vi "SP24_CL_Framework_0.vi"() -> ()   [LabVIEW 2023]
uses:
  <vilib>/Analysis/3filter.llb/Filter Passband Type.ctl
  LVLib/SADI_FW3.lvlib
  <vilib>/ptbypt/NI_PtbyPt.lvlib
  <vilib>/Analysis/NI_AALBase.lvlib
panel:
  in  "Couts/rev":dbl=3704.0
  in  "Tab Control":T1(tab)=enum."Stuff you need to use"
  in  "Latest?":bool=TRUE
  out "SADIs Connected":u32=1
  in  "instance":i32
  in  "Loop Frequency":u16=30000 min=1
  out "MSG CNT":u32=7246531
  in  "Mode Select":T2(ring)=enum."daqMode_pendulum"
  in  "Encoder Pin Location 1":u16(ring)=2 items=["D0"=0, "D1"=1, "D2"=2, "D3"=3, "D4"=4, "D5"=5, "D6"=6, "D8"=8, "D9"=9, "D10"=10, "D11"=11]
  in  "Encoder Pin Location 0":u16(ring) items=["D0"=0, "D1"=1, "D2"=2, "D3"=3, "D4"=4, "D5"=5, "D6"=6, "D8"=8, "D9"=9, "D10"=10, "D11"=11]
  in  "OutputPinMsk":u16=240 format="%x"
  in  "servoEnableMask":u8 format="%x"
  in  "motorEnableMask":u8 format="%x"
  out "Setup Valid":bool=TRUE
  out "Stopped":bool=TRUE
  in  "Output Units":enum16{"Degrees", "Radians"}(ring)
  out "PendEncValMax":u16=500
  in  "ADC GAIN 0":u16(ring)=2 items=["Range_CH_OFF_msk"=0, "Range_pm_10_24_msk"=1, "Range_pm_05_12_msk"=2, "Range_pm_02_56_msk"=3, "Range_pm_01_28_msk"=4, "Range_pm_00_64_msk"=5, "Range_10_24_msk"=9, "Range_05_12_msk"=10, "Range_02_56_msk"=11, "Range_01_28_msk"=12]
  in  "ADC GAIN 3":u16(ring)=2 items=["Range_CH_OFF_msk"=0, "Range_pm_10_24_msk"=1, "Range_pm_05_12_msk"=2, "Range_pm_02_56_msk"=3, "Range_pm_01_28_msk"=4, "Range_pm_00_64_msk"=5, "Range_10_24_msk"=9, "Range_05_12_msk"=10, "Range_02_56_msk"=11, "Range_01_28_msk"=12]
  in  "ADC GAIN 2":u16(ring)=2 items=["Range_CH_OFF_msk"=0, "Range_pm_10_24_msk"=1, "Range_pm_05_12_msk"=2, "Range_pm_02_56_msk"=3, "Range_pm_01_28_msk"=4, "Range_pm_00_64_msk"=5, "Range_10_24_msk"=9, "Range_05_12_msk"=10, "Range_02_56_msk"=11, "Range_01_28_msk"=12]
  in  "ADC GAIN 1":u16(ring)=2 items=["Range_CH_OFF_msk"=0, "Range_pm_10_24_msk"=1, "Range_pm_05_12_msk"=2, "Range_pm_02_56_msk"=3, "Range_pm_01_28_msk"=4, "Range_pm_00_64_msk"=5, "Range_10_24_msk"=9, "Range_05_12_msk"=10, "Range_02_56_msk"=11, "Range_01_28_msk"=12]
  out "FT_ERROR_ENUM":T3(ring)=enum."FT_INVALID_HANDLE"
  out "Loop Time (ms)":dbl=0.48749999950814527 format="%.6f"
  in  "Encoder Resolution 0":u16=360
  in  "Encoder Resolution 1":u16=360
  out "PendEncValMin":u16=10000
  out "Software Version":dbl=3.024 format="%_6g"
  out "Firmware Version":sgl=3.41
  out "Motor Rotation Counts":i32=31626
  out "Motor Velocity":i32=5788
  in  "Cutoff freq: fl":dbl=40.0 format="%0.3f"
  in  "Sampling freq: fs":dbl=2000.0
  in  "initialize":bool
  out "Filtered Platen Rotation Angle":dbl=3294.999499487255 format="%0.2f"
  out "Platen Velocity":dbl=-3.1364198416679514
  out "Total Angle":dbl=3295.4967602591796
  in  "Zero":bool
  in  "Amplitude":dbl=350.0
  in  "Turn On Command":dbl=65.0
  in  "Frequency":dbl=20.0
  in  "Sine (L)/Square (R)":bool
  in  "Enable Motor":bool=TRUE
  in  "Stop":bool=TRUE
  in  "Desired Loop \nTime (ms)":dbl=0.5
  out "Actual Loop \nTime (ms)":dbl=0.500105999999505
  out "Elapsed \nTime (s)":dbl=241.6297153000005
  out "Segments Saved":u32=1
  in  "Save Data?":bool
  out "Platen Rotation Graph":dbl[](graph)=[3294.999499487255]
  out "Platen Vel Graph":dbl[](graph)=[-3.1364198416679514]
  out "Command Signal Graph":dbl[](graph)=[-176.84915368007944]
  out "Command Signal":dbl=-176.84915368007944
  out "Read Call Error Out":u16(ring)=32768 items=["SADI_RESET (FT_OK)"=0, "FT_INVALID_HANDLE"=1, "FT_DEVICE_NOT_FOUND"=2, "FT_DEVICE_NOT_OPENED"=3, "FT_IO_ERROR"=4, "FT_INSUFFICIENT_RESOURCES"=5, "FT_OTHER_ERROR"=18, "FT_NOT_SUPPORTED"=17, "DATA_RECEIVED"=32768, "NO_DATA_AVAIL"=32769, "NO_SADI"=32770]
  out "SADI State":T4(ring)=enum."Run_state"
  # "Platen Rotation & Velocity"
  # "Signal Generator"
  # "Butterworth Filter Settings"
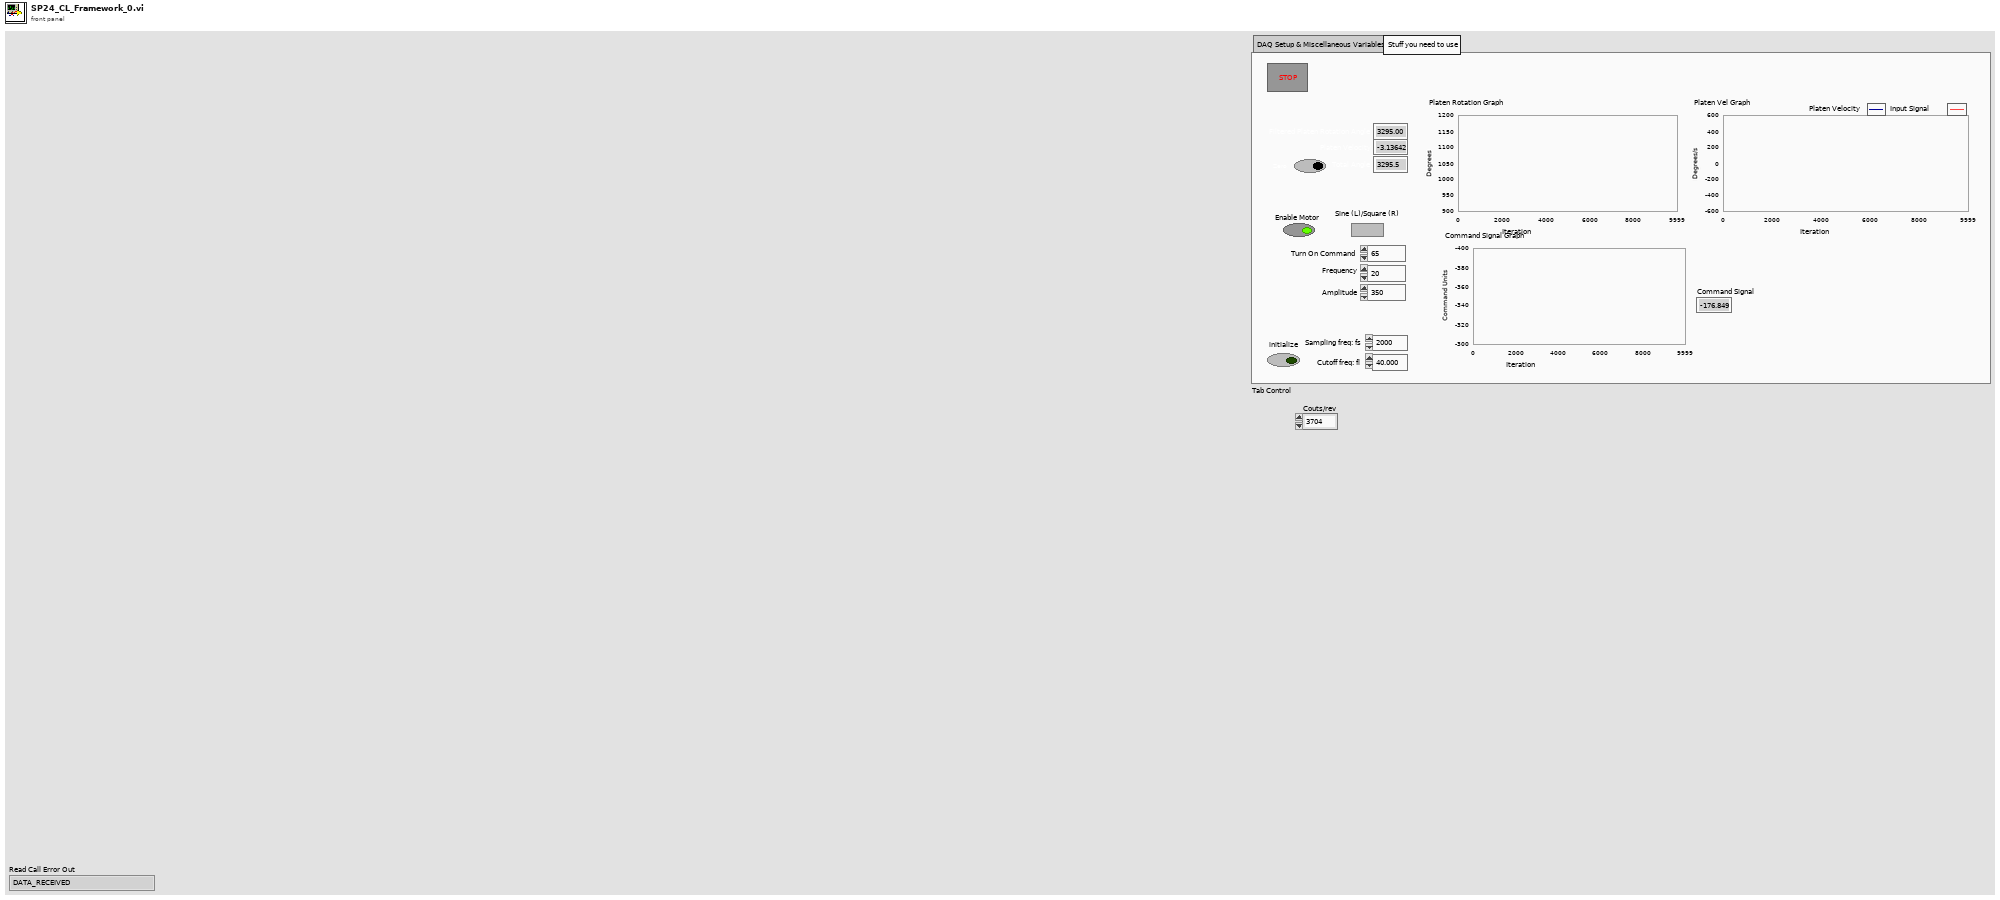
[diagram p1: front panel]
types:
  T1 = enum32{"DAQ Setup & Miscellaneous Variables", "Stuff you need to use"}
  T2 = enum16{"daqMode_unassigned", "daqMode_generic", "daqMode_pendulum", "daqMode_mom"}
  T3 = enum32{"FT_OK", "FT_INVALID_HANDLE", "FT_DEVICE_NOT_FOUND", "FT_DEVICE_NOT_OPENED", "FT_IO_ERROR", "FT_INSUFFICIENT_RESOURCES", "FT_INVALID_PARAMETER", "FT_INVALID_BAUD_RATE", "FT_DEVICE_NOT_OPENED_FOR_ERASE", "FT_DEVICE_NOT_OPENED_FOR_WRITE", "FT_FAILED_TO_WRITE_DEVICE", "FT_EEPROM_READ_FAILED", "FT_EEPROM_WRITE_FAILED", "FT_EEPROM_ERASE_FAILED", "FT_EEPROM_NOT_PRESENT", "FT_EEPROM_NOT_PROGRAMMED", "FT_INVALID_ARGS", "FT_NOT_SUPPORTED", "FT_OTHER_ERROR", "FT_DEVICE_LIST_NOT_READY"}
  T4 = enum32{"NotOpened_state", "Opened_state", "Ready_state", "Setup_state", "InitSent_state", "Start_initiated_state", "Run_state", "StopInitiated_state", "Stopped_state"}
  T5 = typedef "NI_AALBase.lvlib/Filter Passband Type.ctl" = enum32{"Lowpass", "Highpass", "Bandpass", "Bandstop"}
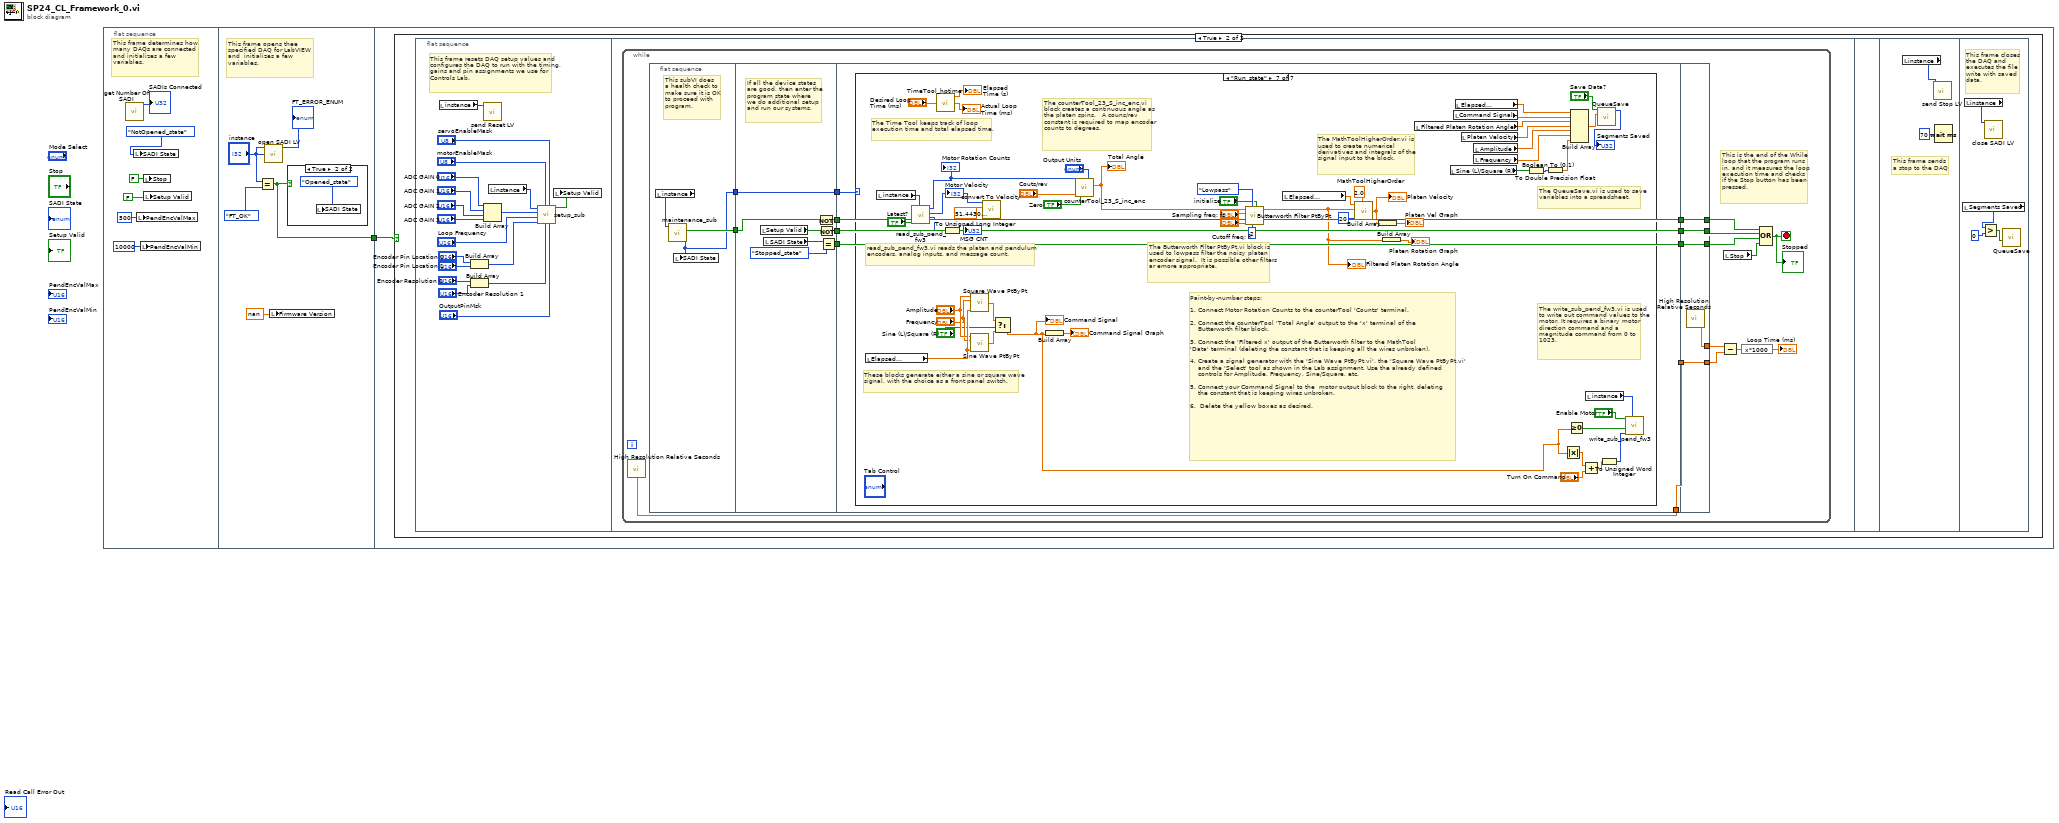
[diagram p0: block diagram]
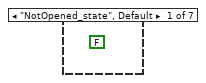
[diagram p4: hidden frame]
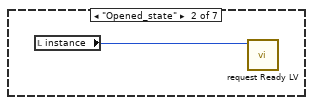
[diagram p5: hidden frame]
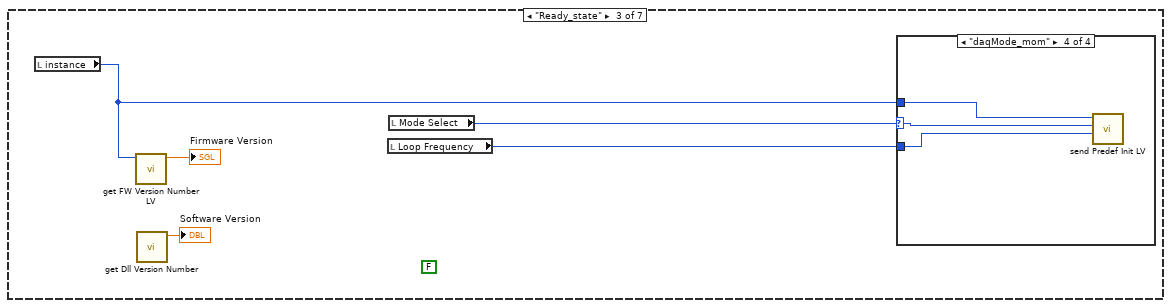
[diagram p6: hidden frame]
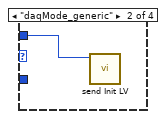
[diagram p8: hidden frame]
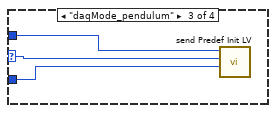
[diagram p9: hidden frame]
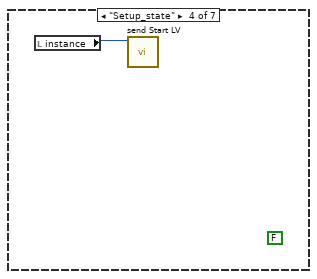
[diagram p10: hidden frame]
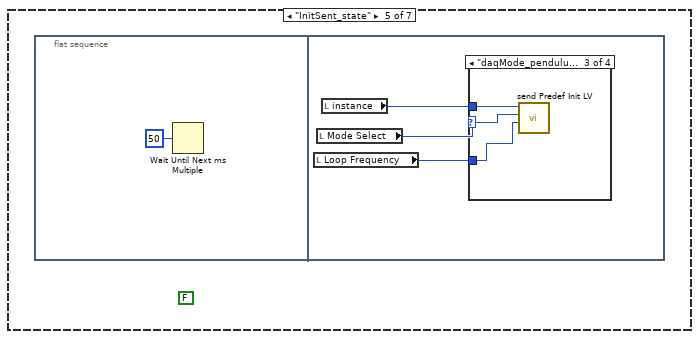
[diagram p11: hidden frame]
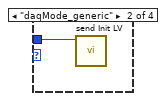
[diagram p13: hidden frame]
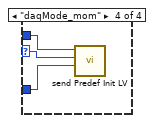
[diagram p14: hidden frame]
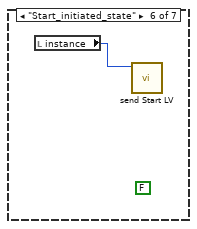
[diagram p15: hidden frame]
diagram:
  n1 = flat-sequence {
    tunnel: [w10] -> w1
    tunnel: w1 -> [w14]
    frame #0 {
      # "This frame determines how many DAQs are connected and initializes a few variables."
      n2 = call "get Number Of SADI.vi"() -> ("function return"=→"SADIs Connected":u32)  [unwired: 11 in]
      n3 = local write "SADI State"(T4."NotOpened_state" ("SADI State")) -> ()
      n4 = local write "PendEncValMax"(u16 500 ("PendEncValMax")) -> ()
      n5 = local write "PendEncValMin"(u16 10000 ("PendEncValMin")) -> ()
      n6 = local write "Stop"(FALSE ("Stop")) -> ()
      n7 = local write "Setup Valid"(FALSE ("Setup Valid")) -> ()
    }
    frame #1 {
      # "This frame opens thee specified DAQ for LabVIEW and  initializes a few variables."
      n8 = Equal?(x="instance", y=T3."FT_OK" ("FT_ERROR_ENUM 2")) -> (x = y?=w10:bool)
      n9 = call "open SADI LV.vi"("deviceNumber"="instance", "instance"="instance") -> ("function return"=→"FT_ERROR_ENUM":u32)  [unwired: 9 in]
      n10 = local write "Firmware Version"(nan ("Firmware Version")) -> ()
      n11 = case shown="True" w10 {
        frame False {
        }
        frame True {
          n12 = local write "SADI State"(T4."Opened_state" ("SADI State 2")) -> ()
        }
      }
    }
    frame #2 {
      n13 = case shown="True" w14 {
        frame False {
        }
        frame True {
          n14 = flat-sequence {
            frame #0 {
              # "This frame resets DAQ setup values and configures the DAQ to run with the timing, gains and pin assignments we use for Controls Lab."
              n15 = local read "instance"() -> (w16:i32)
              n16 = Build Array("Encoder Pin Location 0", "Encoder Pin Location 1") -> (w26:u16[])
              n17 = Build Array("Encoder Resolution 0", "Encoder Resolution 1") -> (w23:u16[])
              n18 = Build Array("ADC GAIN 0", "ADC GAIN 1", "ADC GAIN 2", "ADC GAIN 3") -> (w28:u16[])
              n19 = call "send Reset LV.vi"("instance"=w16) -> ()  [unwired: 11 in]
              n20 = local read "instance"() -> (w17:i32)
              n21 = call "setup_sub.vi"("OutputPinMsk"="OutputPinMsk", "servoEnableMask"="servoEnableMask", "ENC_RES_Array"=w23, "motorEnableMask"="motorEnableMask", "pinLocation_Array"=w26, "Loop Frequency"="Loop Frequency", "ADC_Settings"=w28, "instance"=w17) -> ("Success?"=w18:bool)  [unwired: 3 in]
              n22 = local write "Setup Valid"(w18) -> ()
            }
            frame #1 {
              n23 = while {
                stop <- w47 stop-if-true
                # "This is the end of the While \nloop that the program runs\nin, and it measures the loop\nexecution time and checks\nif the Stop button has been\npressed."
                n24 = call <vilib>:"High Resolution Relative Seconds.vi"() -> ("relative seconds"=w35:dbl)
                n25 = flat-sequence {
                  tunnel: [w55] -> w52
                  tunnel: [w53] -> w33
                  tunnel: w52 -> [w60]
                  tunnel: [w59] -> w46
                  tunnel: [w58] -> w45
                  tunnel: [w57] -> w44
                  tunnel: [w56] -> w34
                  tunnel: w33 -> [w56]
                  tunnel: w46 -> [w68]
                  tunnel: w45 -> [w67]
                  tunnel: w44 -> [w66]
                  tunnel: [w68] -> w43
                  tunnel: [w67] -> w42
                  tunnel: [w66] -> w41
                  tunnel: [w65] -> w39
                  tunnel: w35 -> [w65]
                  tunnel: w34 -> [w64]
                  tunnel: [w150] -> w49
                  tunnel: [w151] -> w50
                  tunnel: [w152] -> w51
                  tunnel: w43 -> [w152]
                  tunnel: w42 -> [w151]
                  tunnel: w41 -> [w150]
                  tunnel: [w149] -> w40
                  tunnel: w39 -> [w148]
                  tunnel: [w148] -> w38
                  frame #0 {
                    # "This subVI does\na health check to\nmake sure it is OK\nto proceed with\nprogram."
                    n26 = local read "instance"() -> (w54:i32)
                    n27 = call "maintenance_sub.vi"("Instance"=w54) -> ("SADI State"=w53:T4, "FT_OK?"=w55:bool)  [unwired: 8 in, 1 out]
                    n28 = local write "SADI State"(w53) -> ()
                  }
                  frame #1 {
                    # "If all the device states\nare good, then enter the\nprogram state where\nwe do additional setup\nand run our systems."
                    n29 = local read "Setup Valid"() -> (w63:bool)
                    n30 = local read "SADI State"() -> (w61:T4)
                    n31 = Not(x=w60) -> (.not. x?=w59:bool)
                    n32 = Not(x=w63) -> (.not. x?=w58:bool)
                    n33 = Equal?(x=w61, y=T4."Stopped_state") -> (x = y?=w57:bool)
                  }
                  frame #2 {
                    n34 = case shown="\"Run_state\"" w64 {
                      frame "NotOpened_state", Default {
                        (unwired) FALSE ("dataToRead?")
                      }
                      frame "Opened_state" {
                        n35 = local read "instance"() -> (w69:i32)
                        n36 = call "request Ready LV.vi"("instance"=w69) -> ()  [unwired: 11 in]
                      }
                      frame "Ready_state" {
                        (unwired) FALSE ("dataToRead?")
                        n37 = local read "instance"() -> (w72:i32)
                        n38 = call "get FW Version Number LV.vi"("instance"=w72) -> ("function return"=→"Firmware Version":dbl)  [unwired: 10 in]
                        n39 = call "get Dll Version Number.vi"() -> ("function return"=→"Software Version":dbl)  [unwired: 11 in]
                        n40 = local read "Loop Frequency"() -> (w70:u16)
                        n41 = local read "Mode Select"() -> (w71:T2)
                        n42 = case shown="\"daqMode_mom\"" w71 {
                          selector: w71 -> [_ _ w77 w80]
                          tunnel: w72 -> [_ w75 w78 w81]
                          tunnel: w70 -> [_ _ w76 w79]
                          frame "daqMode_unassigned", Default {
                          }
                          frame "daqMode_generic" {
                            n43 = call "send Init LV.vi"("instance"=w75) -> ()  [unwired: 11 in]
                          }
                          frame "daqMode_pendulum" {
                            n44 = call "send Predef Init LV.vi"("freq"=w76, "selection"=w77, "instance"=w78) -> ()  [unwired: 9 in]
                          }
                          frame "daqMode_mom" {
                            n45 = call "send Predef Init LV.vi"("freq"=w79, "selection"=w80, "instance"=w81) -> ()  [unwired: 9 in]
                          }
                        }
                      }
                      frame "Setup_state" {
                        (unwired) FALSE ("dataToRead?")
                        n46 = local read "instance"() -> (w82:i32)
                        n47 = call "send Start LV.vi"("instance"=w82) -> ()  [unwired: 11 in]
                      }
                      frame "InitSent_state" {
                        (unwired) FALSE ("dataToRead?")
                        n48 = flat-sequence {
                          frame #0 {
                            n49 = Wait Until Next ms Multiple(millisecond multiple=u32 50) -> ()  [unwired: 1 out]
                          }
                          frame #1 {
                            n50 = local read "Loop Frequency"() -> (w84:u16)
                            n51 = local read "Mode Select"() -> (w85:T2)
                            n52 = local read "instance"() -> (w86:i32)
                            n53 = case shown="\"daqMode_pendulum\"" w85 {
                              selector: w85 -> [_ _ w90 w92]
                              tunnel: w86 -> [_ w87 w89 w93]
                              tunnel: w84 -> [_ _ w88 w91]
                              frame "daqMode_unassigned", Default {
                              }
                              frame "daqMode_generic" {
                                n54 = call "send Init LV.vi"("instance"=w87) -> ()  [unwired: 11 in]
                              }
                              frame "daqMode_pendulum" {
                                n55 = call "send Predef Init LV.vi"("freq"=w88, "selection"=w90, "instance"=w89) -> ()  [unwired: 9 in]
                              }
                              frame "daqMode_mom" {
                                n56 = call "send Predef Init LV.vi"("freq"=w91, "selection"=w92, "instance"=w93) -> ()  [unwired: 9 in]
                              }
                            }
                          }
                        }
                      }
                      frame "Start_initiated_state" {
                        (unwired) FALSE ("dataToRead?")
                        n57 = local read "instance"() -> (w94:i32)
                        n58 = call "send Start LV.vi"("instance"=w94) -> ()  [unwired: 11 in]
                      }
                      frame "Run_state" {
                        # "Paint-by-number steps:\n\n1. Connect Motor Rotation Counts to the counterTool 'Counts' terminal.\n\n2. Connect the counterTool 'Total Angle' output to the 'x' terminal of the \n    Butterworth filter block.\n\n3. Connect the 'FIltered x' output of the Butterworth filter to the MathTool \n'Data' terminal (deleting the constant that is keeping all the wires unbroken).\n\n4. Create a signal generator with the 'Sine Wave PtByPt.vi', the 'Square Wave PtByPt.vi'\n    and the 'Select' tool as shown in the Lab assignment. Use the already defined\n    controls for Amplitude, Frequency, Sine/Square, etc.\n\n5. Connect your Command Signal to the  motor output block to the right, deleting\n    the constant that is keeping wires unbroken.\n\n6.  Delete the yellow boxes as desired."
                        # "The counterTool_23_S_inc_enc.vi block creates a continuous angle as the platen spins.   A couns/rev constant is required to map encoder counts to degrees."
                        # "The write_sub_pend_fw3.vi is used to write out command values to the motor. It requires a binary motor direction command and a magnitude command from 0 to 1023."
                        # "The QueueSave.vi is used to save variables into a spreadsheet."
                        # "The MathToolHigherOrder.vi is used to create numerical derivatives and integrals of the signal input to the block."
                        # "The Butterworth Filter PtByPt.vi block is used to lowpass filter the noisy platen encoder signal.  It is possible other filters ar emore appropriate."
                        # "These blocks generate either a sine or square wave signal, with the choice as a front panel switch."
                        # "read_sub_pend_fw3.vi reads the platen and pendulum encoders, analog inputs, and message count."
                        # "The Time Tool keeps track of loop execution time and total elapsed time."
                        n59 = local read "Elapsed \nTime (s)"() -> (w100:dbl)
                        n60 = local read "instance"() -> (w145:i32)
                        n61 = call "read_sub_pend_fw3.vi"("instance"=w145, "Latest?"="Latest?") -> ("MSG CNT"=w143:u32, "ENC VEL 0"=w110:u16, "ENC POS 0"=w102:i32)  [unwired: 6 in, 1 out]
                        "Motor Velocity" <- w110
                        "Motor Rotation Counts" <- w102
                        n62 = call "TimeTool_hptime.vi"("Desired Loop Time (ms)"="Desired Loop \nTime (ms)") -> ("elapsed time (s)"=→"Elapsed \nTime (s)":dbl, "dt (ms)"=→"Actual Loop \nTime (ms)":dbl)  [unwired: 1 out]
                        n63 = To Unsigned Long Integer(number=w143) -> (unsigned 32bit integer=→"MSG CNT":u32)
                        n64 = call <vilib>:"Square Wave PtByPt.vi"("amplitude"="Amplitude", "frequency"="Frequency", "time"=w100) -> ("square wave"=w97:dbl)  [unwired: 2 in]
                        n65 = call <vilib>:"Sine Wave PtByPt.vi"("time"=w100, "frequency"="Frequency", "amplitude"="Amplitude") -> ("sine wave"=w101:dbl)  [unwired: 1 in]
                        n66 = call "convert To Velocity.vi"("gearRatio"=sgl 51.443, "velVal"=w110) -> ()  [unwired: 9 in, 1 out]
                        n67 = Select(t=w97, s="Sine (L)/Square (R)", f=w101) -> (s? t:f=w95:dbl)
                        "Command Signal" <- w95
                        n68 = Build Array(w95) -> (→"Command Signal Graph":dbl[])
                        n69 = call "counterTool_23_S_inc_enc.vi"("Counts"=w102, "Zero"="Zero", "Couts/rev"="Couts/rev", "Output Units"="Output Units") -> ("Total Angle"=w111:dbl)  [unwired: 3 in, 1 out]
                        "Total Angle" <- w111
                        n70 = call <vilib>:"Butterworth Filter PtByPt.vi"("initialize"="initialize", "order"=2, "filter type"=Filter_Passband_Type."Lowpass", "low cutoff freq: fl"="Cutoff freq: fl", "sampling freq: fs"="Sampling freq: fs", "x"=w111) -> ("Filtered x"=w104:dbl)  [unwired: 3 in, 1 out]
                        "Filtered Platen Rotation Angle" <- w104
                        n71 = local read "Elapsed \nTime (s)"() -> (w134:dbl)
                        n72 = call "MathToolHigherOrder.vi"("Time"=w134, "Interp Order (NaN for Npts-1)"=2.0, "Data"=w104, "n-diff"=20) -> ("1st derivative"=w113:dbl)  [unwired: 2 in, 2 out]
                        "Platen Velocity" <- w113
                        n73 = Build Array(w113) -> (→"Platen Vel Graph":dbl[])
                        n74 = Build Array(w104) -> (→"Platen Rotation Graph":dbl[])
                        n75 = local read "Filtered Platen Rotation Angle"() -> (w122:dbl)
                        n76 = local read "Sine (L)/Square (R)"() -> (w116:bool)
                        n77 = local read "Command Signal"() -> (w123:dbl)
                        n78 = local read "Elapsed \nTime (s)"() -> (w138:dbl)
                        n79 = local read "Platen Velocity"() -> (w121:dbl)
                        n80 = local read "Amplitude"() -> (w119:dbl)
                        n81 = local read "Frequency"() -> (w118:dbl)
                        n82 = Boolean To (0,1)(Boolean=w116) -> (0, 1=w115:i16)
                        n83 = To Double Precision Float(number=w115) -> (double precision float=w117:dbl)
                        n84 = Absolute Value(x=w95) -> (abs(x)=w108:dbl)
                        n85 = Greater Or Equal To 0?(x=w95) -> (x >= 0?=w126:bool)
                        n86 = Build Array "Build Array"(w138, w123, w122, w121, w119, w118, w117) -> (w140:dbl[])
                        n87 = Add(x=w108, y="Turn On Command") -> (x+y=w107:dbl)
                        n88 = local read "instance"() -> (w120:i32)
                        n89 = call "QueueSave.vi"("Data In"=w140, "Save Data?"="Save Data?") -> ("Segments Saved"=→"Segments Saved":u32)  [unwired: 3 in, 2 out]
                        n90 = To Unsigned Word Integer(number=w107) -> (unsigned 16bit integer=w106:u16)
                        n91 = call "write_sub_pend_fw3.vi"("instance"=w120, "pendMotorVal"=w106, "pendDir"=w126, "enableWrite"="Enable Motor") -> ()  [unwired: 8 in]
                      }
                    }
                  }
                  frame #3 {
                    n92 = call <vilib>:"High Resolution Relative Seconds.vi"() -> ("relative seconds"=w149:dbl)
                  }
                }
                n93 = Subtract(x=w40, y=w38) -> (x-y=w37:dbl)
                n94 = local read "Stop"() -> (w48:bool)
                n95 = expression code="x*1000"(w37) -> (→"Loop Time (ms)":dbl)
                n96 = Compound Arithmetic op=OR(w51, w50, w49, w48) -> (w47:bool)
                "Stopped" <- w47
              }
            }
            frame #2 {
            }
            frame #3 {
              # "This frame sends\na stop to the DAQ"
              n97 = local read "instance"() -> (w154:i32)
              n98 = call "send Stop LV.vi"("instance"=w154) -> ()  [unwired: 11 in]
              n99 = Wait (ms)(milliseconds to wait=u32 70) -> ()  [unwired: 1 out]
            }
            frame #4 {
              # "This frame closes\nthe DAQ and \nexecutes the file\nwrite with saved\ndata."
              n100 = local read "Segments Saved"() -> (w157:u32)
              n101 = local read "instance"() -> (w158:i32)
              n102 = Greater?(x=w157, y=u32 0) -> (0:w156:bool)
              n103 = call "close SADI LV.vi"("instance"=w158) -> ()  [unwired: 10 in, 1 out]
              n104 = call "QueueSave.vi"("Write To Spreadsheet"=w156) -> ()  [unwired: 4 in, 3 out]
            }
          }
        }
      }
    }
  }
